vi "sio getbaud.vi"(11 "port":i32) -> (3 "function return":i32)   [LabVIEW 2015, in "PCOMM.lvlib"]
doc: "long WINAPI sio_getbaud(int port);"
uses:
  PCOMM.lvlib
  PCOMM.DLL
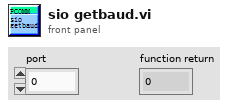
[diagram p1: front panel]
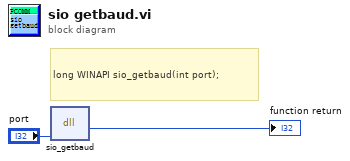
[diagram p0: block diagram]
diagram:
  # "long WINAPI sio_getbaud(int port);"
  n1 = dll-call lib="PTH2^abs EDesktopLabview串口助手串口助手2.0Ing10_v3.2.0SubVIpcomm库PCOMM.*" fn="sio_getbaud"("port"="port") -> (→"function return":i32)  [unwired: 4 in, 2 out]
